vi "_GroupCreate.vi"(2 "error in":errorcluster, 3 "ignored devices":string[](array[string]), 4 "managed devices":string[](array[string]), 5 "group name":string) -> (0 "error out":errorcluster, 1 "group id":i32)   [LabVIEW 2014, in "tango.lvlib"]
uses:
  tango.lvlib
  tango_binding.so
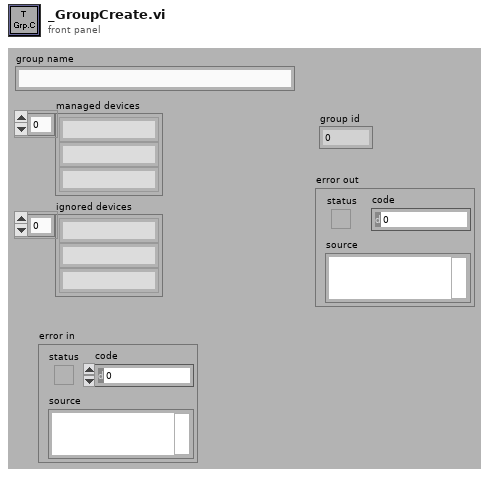
[diagram p1: front panel]
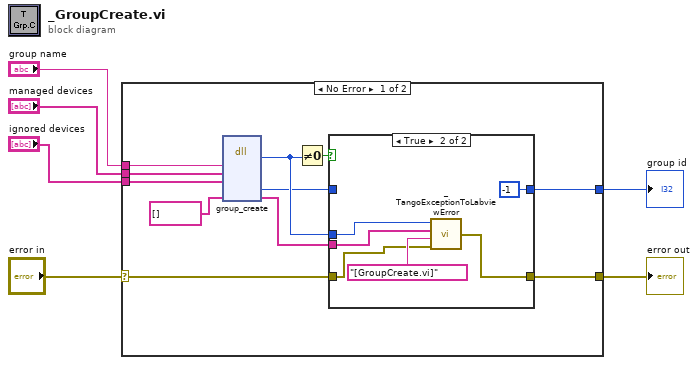
[diagram p0: block diagram]
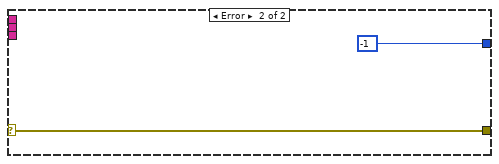
[diagram p3: hidden frame]
diagram:
  n1 = case shown="No Error" "error in" {
    selector: "error in" -> [w12 w27]
    tunnel: "group name" -> [w17 _]
    tunnel: "managed devices" -> [w16 _]
    tunnel: "ignored devices" -> [w15 _]
    tunnel: [w7 -1 ("group_id")] -> w3
    tunnel: [w11 w27] -> w1
    frame No Error {
      n2 = dll-call lib="tango_binding.*" fn="group_create"("group_name"=w17, "managed_devices"=w16, "ignored_devices"=w15, "error_stack"=string[] [] ("error stack")) -> ("return type"=w10:i32, "group_id"=w8:i32, "error_stack"=w9:string[])  [unwired: 7 in, 2 out]
      n3 = Not Equal To 0?(x=w10) -> (x != 0?=w13:bool)
      n4 = case shown="True" w13 {
        tunnel: w12 -> [w19 w20]
        tunnel: [w19 w25] -> w11
        tunnel: w10 -> [_ w22]
        tunnel: w9 -> [_ w23]
        tunnel: w8 -> [w18 _]
        tunnel: [w18 -1 ("group_id")] -> w7
        frame False {
        }
        frame True {
          n5 = call "_TangoExceptionToLabviewError.vi"("error in"=w20, "location"="[GroupCreate.vi]", "error stack"=w23, "error code"=w22) -> ("error out"=w25:errorcluster)
        }
      }
    }
    frame Error {
    }
  }
  "group id" <- w3
  "error out" <- w1
